vi "Ramp Generation.vi"() -> ()   [LabVIEW 2019]
panel:
  out "Ramp Output":waveform(dbl)(graph)
  in  "# Points":dbl
  in  "Time Span (s)":dbl
  in  "Max":dbl
  in  "Min":dbl
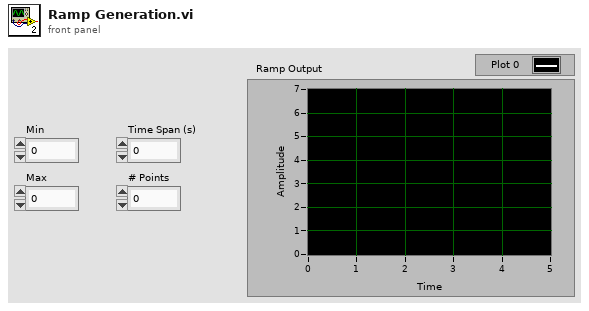
[diagram p1: front panel]
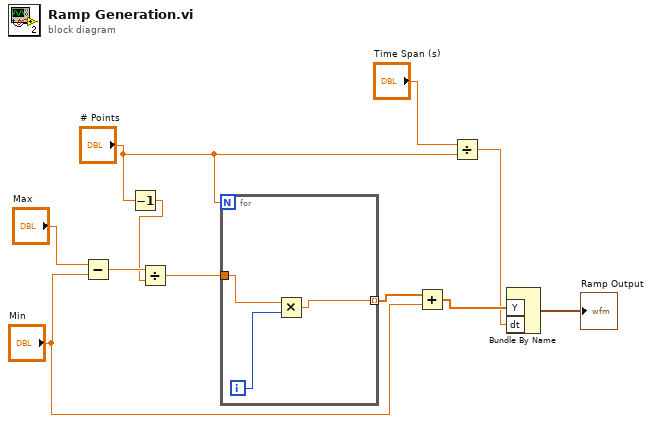
[diagram p0: block diagram]
diagram:
  n1 = Subtract(x="Max", y="Min") -> (x-y=w10:dbl)
  n2 = Decrement(x="# Points") -> (x-1=w9:dbl)
  n3 = Divide(x=w10, y=w9) -> (x/y=w8:dbl)
  n4 = for {
    N: "# Points" -> [_]
    tunnel: w8 -> [w13]
    tunnel: [w12] -> w7 mode=indexing
    i -> [w14]
    n5 = Multiply(x=w13, y=w14) -> (x*y=w12:dbl)
  }
  n6 = Add(x=w7, y="Min") -> (x+y=w4:dbl[])
  n7 = Divide(x="Time Span (s)", y="# Points") -> (x/y=w3:dbl)
  n8 = Bundle By Name("Y"=w4, "dt"=w3) -> (→"Ramp Output":waveform(dbl))  [unwired: 1 in]
